vi "main_2.vi"() -> ()   [LabVIEW 2011]
uses:
  vehicleCluster_2.ctl
panel:
  out "Cluster 2":T1
  out "name":string
  out "numberOfWheels":dbl
  in  "Cluster":T1
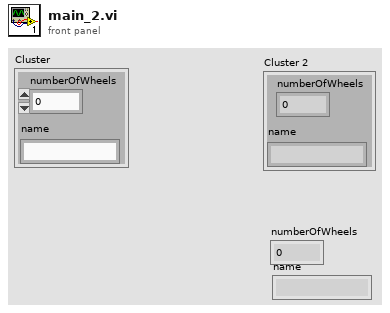
[diagram p1: front panel]
types:
  T1 = typedef "vehicleCluster_2.ctl" = cluster{"numberOfWheels":dbl, "name":string}
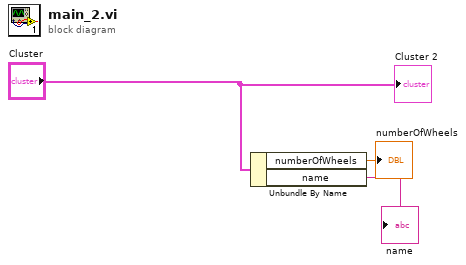
[diagram p0: block diagram]
diagram:
  n1 = Unbundle By Name("Cluster") -> ("numberOfWheels"=→"numberOfWheels":dbl, "name"=→"name":string)
  "Cluster 2" <- "Cluster"
